vi "Password input.vi"() -> (0 "Boolean":bool, 3 "String 2":string)   [LabVIEW 2013]
panel:
  in  "Cancel Button":bool
  in  "OK Button":bool
  in  "Input Password":string
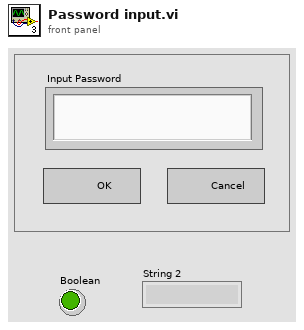
[diagram p1: front panel]
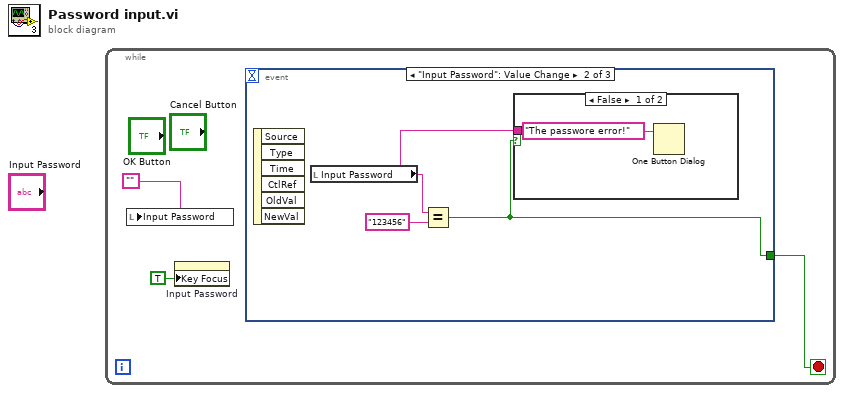
[diagram p0: block diagram]
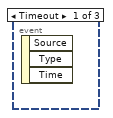
[diagram p2: hidden frame]
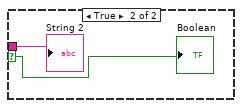
[diagram p3: hidden frame]
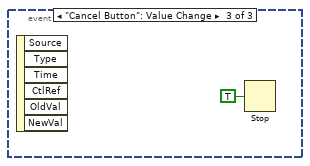
[diagram p4: hidden frame]
diagram:
  n1 = while {
    stop <- w3 stop-if-true
    n2 = local write "Input Password"("") -> ()
    n3 = property on="Input Password" class="Str"("Key Focus"=TRUE) -> ()  [unwired: 2 in, 2 out]
    n4 = event shown="[1] \"Input Password\": Value Change" {
      selector: _ -> [_ _ _]
      dyn-events: _ -> [_ _ _]
      timeout: _ -> [_ _ _]
      tunnel: [_ w5 _] -> w3
      event Timeout {
        n5 = event-data() -> ()  [unwired: 1 in, 3 out]
      }
      event "Input Password": Value Change {
        n6 = event-data() -> ()  [unwired: 1 in, 6 out]
        n7 = local read "Input Password"() -> (w4:string)
        n8 = Equal?(x=w4, y="123456") -> (x = y?=w5:bool)
        n9 = case shown="False" w5 {
          selector: w5 -> [_ w8]
          tunnel: w4 -> [_ w9]
          frame False {
            n10 = One Button Dialog(message="The passwore error!") -> ()  [unwired: 1 in, 1 out]
          }
          frame True {
            "String 2" <- w9
            "Boolean" <- w8
          }
        }
      }
      event "Cancel Button": Value Change {
        n11 = event-data() -> ()  [unwired: 1 in, 6 out]
        n12 = Stop(stop? (T)=TRUE) -> ()
      }
    }
  }
